vi "Explorer_Send_to_SPIKE.vi"(10 "queueName":string="PV_script", 11 "python":string) -> (0 "error out":errorcluster)   [LabVIEW 2022 SP3]
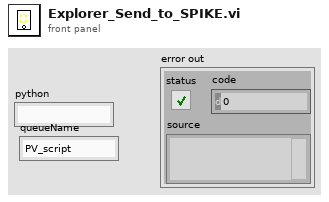
[diagram p1: front panel]
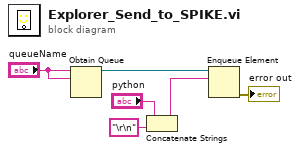
[diagram p0: block diagram]
diagram:
  n1 = Obtain Queue(name (unnamed)="queueName", element data type="queueName") -> (queue out=w3:refnum<queue>)  [unwired: 3 in, 2 out]
  n2 = Concatenate Strings("python", "\r\n" ("string")) -> (w6:string)
  n3 = Enqueue Element(queue=w3, element=w6) -> (error out=→"error out":errorcluster)  [unwired: 2 in, 2 out]
